vi "LINX - Digital Write N Channels.vi"() -> ()   [LabVIEW 2020]
doc: "This example demonstrates how to write N channels of digital ouput from a LINX device."
uses:
  vi.lib/MakerHub/LINX/Public/Peripherals/Digital/Digital Write N Chans.vi
  vi.lib/MakerHub/LINX/Private/Local IO/LinxDigitalWrite.vi
  vi.lib/MakerHub/LINX/Public/Utilities/Check Channel.vi
  vi.lib/MakerHub/LINX/Public/Utilities/Open Serial.vi
  vi.lib/MakerHub/LINX/Private/Utilties/Generate Error.vi
  vi.lib/MakerHub/LINX/LMH-LINX.lvlib
panel:
  in  "Values":bool[](array[boolean])=[FALSE, FALSE, FALSE, FALSE]
  in  "D0 Channels":u8[](array[numeric])=[2, 3, 4, 5]
  in  "Stop Button":bool
  in  "Serial Port":refnum<visa-resource-name>
  # "LINX Device Settings"
  # "DO Values"
  # "Digital Write N Channel Example\n\nThis example demonstrates how to write multiple digital output channels.\n\nInstructions\n1. Select the COM Port associated with the LINX Device.\n2. Select the DO Channels to write.\n3. Click the Run Arrow."
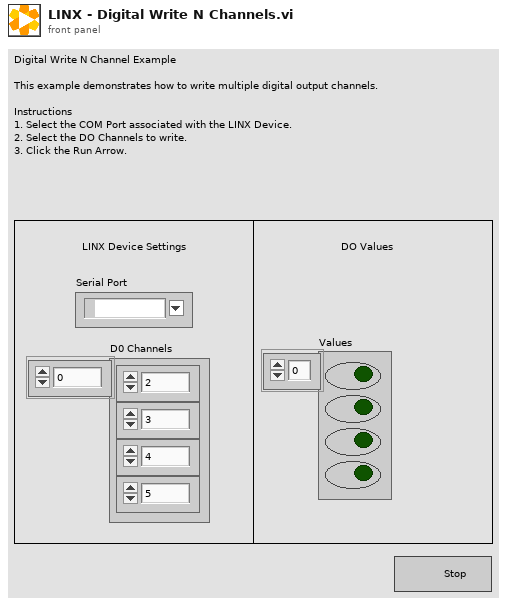
[diagram p1: front panel]
types:
  T1 = typedef "LMH-LINX.lvlib/LINX Ref.ctl" = cluster{"IO":T2, "Interface":T3, "LINX Device Config":T4}
  T2 = typedef "LMH-LINX.lvlib/Platform.ctl" = enum16{"Remote", "Local"}
  T3 = typedef "LMH-LINX.lvlib/Interface.ctl" = enum16{"Serial", "TCP"}
  T4 = typedef "Device.lvlib/LINX Device Config.ctl" = cluster{"Interface":T3, "COM Port":refnum<visa-resource-name>, "TCP Configuration":T5, "Device Family":u8, "Device ID":u8, "Device Name":string, "TCP Ref":refnum<k5>, "Channels":T6}
  T5 = typedef "Device.lvlib/TCP Config.ctl" = cluster{"IP Address":string, "Port":u16}
  T6 = typedef "LMH-LINX.lvlib/Channels.ctl" = cluster{"DI":u8[], "DO":u8[], "AI":u8[], "AO":u8[], "PWM":u8[], "QE":u8[], "UART":u8[], "I2C 2":u8[], "SPI":u8[], "CAN":u8[], "Servo":u8[], "AI Ref (V)":dbl, "AI Resolution (Bits)":u8, "AO Ref (V)":dbl, "AO Resolution (Bits)":u8}
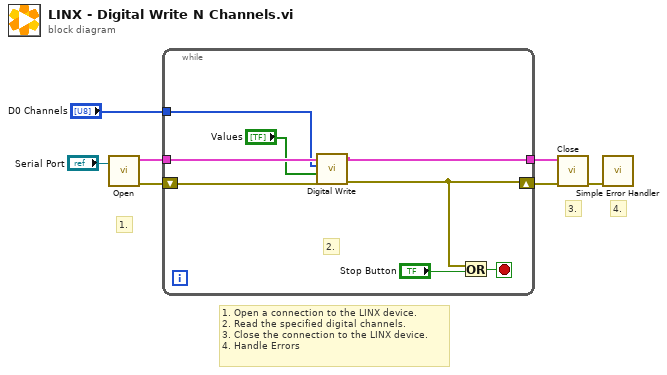
[diagram p0: block diagram]
diagram:
  # "1. Open a connection to the LINX device.\n2. Read the specified digital channels.\n3. Close the connection to the LINX device.\n4. Handle Errors"
  # "4."
  # "3."
  # "1."
  n1 = call-poly "Open.vi"("Serial Port"="Serial Port") -> ("Error Out"=w6:errorcluster, "LINX Resource"=w7:T1)  [unwired: 8 in, 1 out]
  n2 = while {
    tunnel: w7 -> [w11]
    tunnel: [w12] -> w5
    shift-right: [w13] -> w4
    shift-left: w6 -> [w10]
    tunnel: "D0 Channels" -> [w9]
    stop <- w15 stop-if-true
    # "2."
    n3 = call-poly "Digital Write.vi"("Error In"=w10, "Values"="Values", "DO Channels"=w9, "LINX Resource"=w11) -> ("Error Out"=w13:errorcluster, "LINX Resource"=w12:T1)  [unwired: 6 in]
    n4 = Or(x=w13, y="Stop Button") -> (x .or. y?=w15:bool)
  }
  n5 = call "Close.vi"("Error In"=w4, "LINX Resource"=w5) -> ("Error Out"=w2:errorcluster)  [unwired: 9 in]
  n6 = call <vilib>:"Simple Error Handler.vi"("error in (no error)"=w2) -> ()  [unwired: 4 in, 5 out]
